vi "RNG.vi"() -> ()   [LabVIEW 2014]
panel:
  out "RNG'd Number":dbl
  in  "MaxValue":dbl
  in  "MinValue":dbl
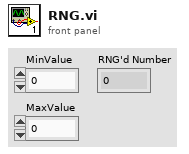
[diagram p1: front panel]
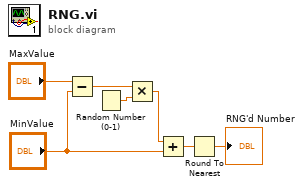
[diagram p0: block diagram]
diagram:
  n1 = Subtract(x="MaxValue", y="MinValue") -> (x-y=w6:dbl)
  n2 = Random Number (0-1)() -> (number: 0 to 1=w5:dbl)
  n3 = Multiply(x=w6, y=w5) -> (x*y=w4:dbl)
  n4 = Add(x=w4, y="MinValue") -> (x+y=w2:dbl)
  n5 = Round To Nearest(number=w2) -> (nearest integer value=→"RNG'd Number":dbl)
